vi "SudokuSolver.vi"() -> ()   [LabVIEW 2010]
uses:
  SudukuBoard/SudokuBoard.lvclass
  Graph/Graph.lvclass
panel:
  in  "Exit":bool
  in  "Solve":bool
  in  "Ultimate":bool
  in  "Hard":bool
  in  "Medium":bool
  in  "Easy":bool
  out "Board":T1(array[cluster])
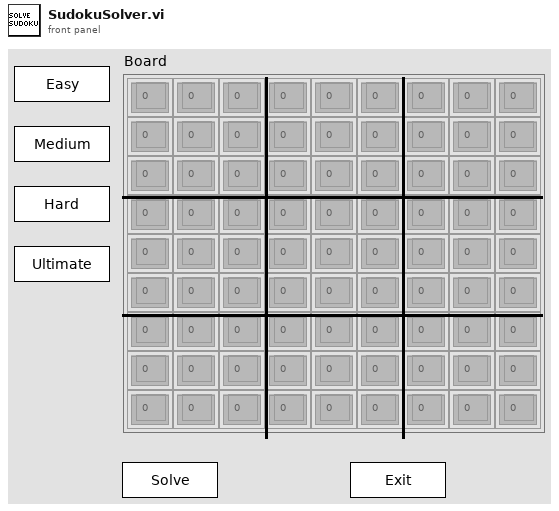
[diagram p1: front panel]
types:
  T1 = cluster{"dimension size":i32, "dimension size 2":bool}[][]
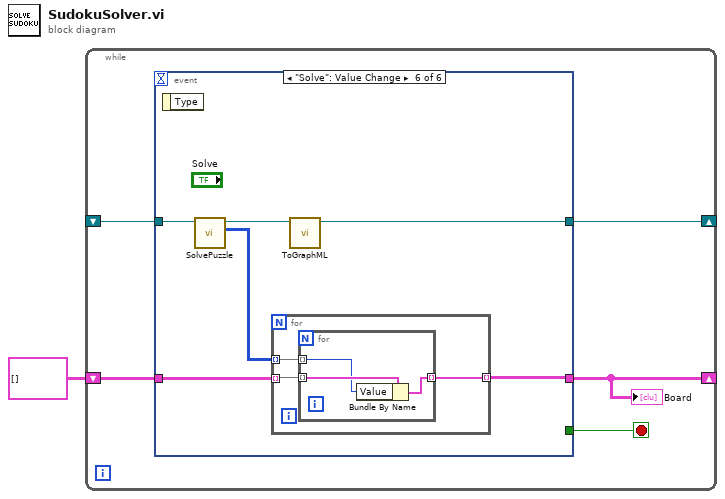
[diagram p0: block diagram]
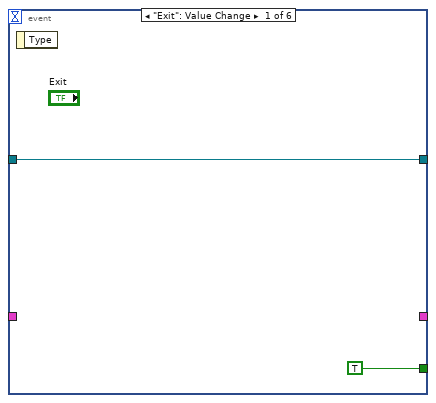
[diagram p2: hidden frame]
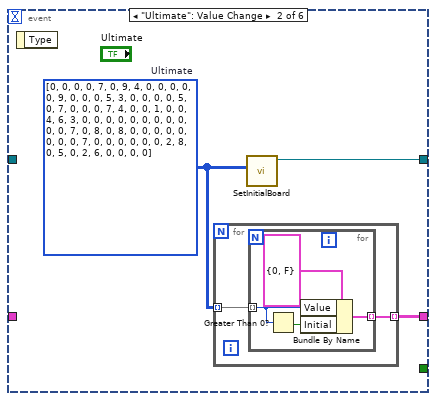
[diagram p3: hidden frame]
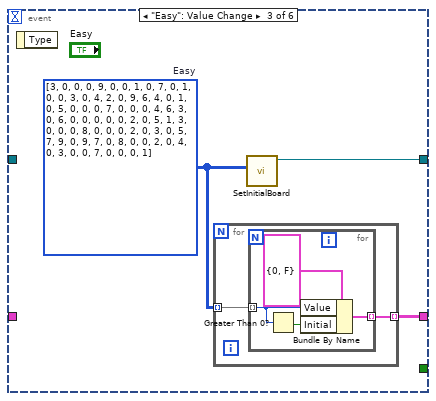
[diagram p4: hidden frame]
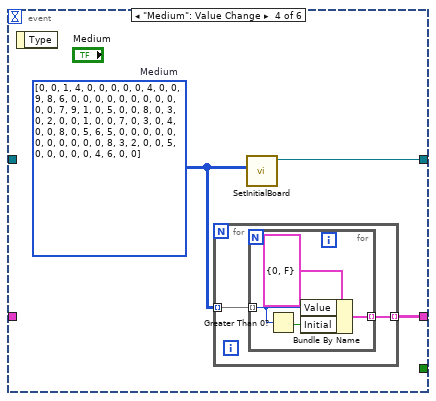
[diagram p5: hidden frame]
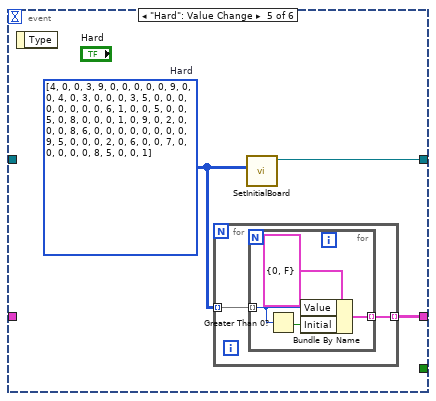
[diagram p6: hidden frame]
diagram:
  n1 = while {
    shift-right: [w5] -> _
    shift-left: _ -> [w4]
    shift-right: [w3] -> _
    shift-left: cluster{"Value":i32, "Initial":bool}[][] [] -> [w2]
    stop <- w6 stop-if-true
    n2 = event shown="[5] \"Solve\": Value Change" {
      selector: _ -> [_ _ _ _ _ _]
      dyn-events: _ -> [_ _ _ _ _ _]
      timeout: _ -> [_ _ _ _ _ _]
      tunnel: [TRUE _ _ _ _ _] -> w6
      tunnel: [w7 w11 w20 w29 w38 w45] -> w5
      tunnel: w4 -> [w7 _ _ _ _ w50]
      tunnel: [_ w9 w18 w28 w36 w47] -> w3
      tunnel: w2 -> [_ _ _ _ _ w49]
      event "Exit": Value Change {
        n3 = event-data() -> ()  [unwired: 1 in, 1 out]
      }
      event "Ultimate": Value Change {
        w10 = i32[][] [[0, 0, 0, 0, 7, 0, 9, 4, 0], [0, 0, 0, 0, 9, 0, 0, 0, 5], [3, 0, 0, 0, 0, 5, 0, 7, 0], [0, 0, 7, 4, 0, 0, 1, 0, 0], [4, 6, 3, 0, 0, 0, 0, 0, 0], [0, 0, 0, 0, 0, 7, 0, 8, 0], [8, 0, 0, 0, 0, 0, 0, 0, 0], [7, 0, 0, 0, 0, 0, 0, 2, 8], [0, 5, 0, 2, 6, 0, 0, 0, 0]]  # Ultimate
        n4 = event-data() -> ()  [unwired: 1 in, 1 out]
        n5 = for {
          tunnel: w10 -> [w13] mode=indexing
          tunnel: [w12] -> w9 mode=indexing
          n6 = for {
            tunnel: w13 -> [w16] mode=indexing
            tunnel: [w17] -> w12 mode=indexing
            n7 = Greater Than 0?(x=w16) -> (x > 0?=w14:bool)
            n8 = Bundle By Name(cluster=cluster{"Value":i32, "Initial":bool} {"Value"=0, "Initial"=FALSE} ("Cell"), "Value"=w16, "Initial"=w14) -> (w17:cluster{"Value":i32, "Initial":bool})
          }
        }
        n9 = call "SetInitialBoard.vi"("InitialBoard"=w10) -> ("SudukuBoard out"=w11:refnum<class "SudokuBoard.lvclass">)  [unwired: 9 in, 1 out]
      }
      event "Easy": Value Change {
        w19 = i32[][] [[3, 0, 0, 0, 9, 0, 0, 1, 0], [7, 0, 1, 0, 0, 3, 0, 4, 2], [0, 9, 6, 4, 0, 1, 0, 5, 0], [0, 0, 7, 0, 0, 0, 4, 6, 3], [0, 6, 0, 0, 0, 0, 0, 2, 0], [5, 1, 3, 0, 0, 0, 8, 0, 0], [0, 2, 0, 3, 0, 5, 7, 9, 0], [9, 7, 0, 8, 0, 0, 2, 0, 4], [0, 3, 0, 0, 7, 0, 0, 0, 1]]  # Easy
        n10 = event-data() -> ()  [unwired: 1 in, 1 out]
        n11 = for {
          tunnel: w19 -> [w22] mode=indexing
          tunnel: [w21] -> w18 mode=indexing
          n12 = for {
            tunnel: w22 -> [w25] mode=indexing
            tunnel: [w26] -> w21 mode=indexing
            n13 = Greater Than 0?(x=w25) -> (x > 0?=w23:bool)
            n14 = Bundle By Name(cluster=cluster{"Value":i32, "Initial":bool} {"Value"=0, "Initial"=FALSE} ("Cell"), "Value"=w25, "Initial"=w23) -> (w26:cluster{"Value":i32, "Initial":bool})
          }
        }
        n15 = call "SetInitialBoard.vi"("InitialBoard"=w19) -> ("SudukuBoard out"=w20:refnum<class "SudokuBoard.lvclass">)  [unwired: 9 in, 1 out]
      }
      event "Medium": Value Change {
        w27 = i32[][] [[0, 0, 1, 4, 0, 0, 0, 0, 0], [4, 0, 0, 9, 8, 6, 0, 0, 0], [0, 0, 0, 0, 0, 0, 0, 0, 7], [9, 1, 0, 5, 0, 0, 8, 0, 3], [0, 2, 0, 0, 1, 0, 0, 7, 0], [3, 0, 4, 0, 0, 8, 0, 5, 6], [5, 0, 0, 0, 0, 0, 0, 0, 0], [0, 0, 0, 8, 3, 2, 0, 0, 5], [0, 0, 0, 0, 0, 4, 6, 0, 0]]  # Medium
        n16 = event-data() -> ()  [unwired: 1 in, 1 out]
        n17 = for {
          tunnel: w27 -> [w31] mode=indexing
          tunnel: [w30] -> w28 mode=indexing
          n18 = for {
            tunnel: w31 -> [w34] mode=indexing
            tunnel: [w35] -> w30 mode=indexing
            n19 = Greater Than 0?(x=w34) -> (x > 0?=w32:bool)
            n20 = Bundle By Name(cluster=cluster{"Value":i32, "Initial":bool} {"Value"=0, "Initial"=FALSE} ("Cell"), "Value"=w34, "Initial"=w32) -> (w35:cluster{"Value":i32, "Initial":bool})
          }
        }
        n21 = call "SetInitialBoard.vi"("InitialBoard"=w27) -> ("SudukuBoard out"=w29:refnum<class "SudokuBoard.lvclass">)  [unwired: 9 in, 1 out]
      }
      event "Hard": Value Change {
        w37 = i32[][] [[4, 0, 0, 3, 9, 0, 0, 0, 0], [0, 9, 0, 0, 4, 0, 3, 0, 0], [0, 3, 5, 0, 0, 0, 0, 0, 0], [0, 0, 6, 1, 0, 0, 5, 0, 0], [5, 0, 8, 0, 0, 0, 1, 0, 9], [0, 2, 0, 0, 0, 8, 6, 0, 0], [0, 0, 0, 0, 0, 0, 9, 5, 0], [0, 0, 2, 0, 6, 0, 0, 7, 0], [0, 0, 0, 0, 8, 5, 0, 0, 1]]  # Hard
        n22 = event-data() -> ()  [unwired: 1 in, 1 out]
        n23 = for {
          tunnel: w37 -> [w40] mode=indexing
          tunnel: [w39] -> w36 mode=indexing
          n24 = for {
            tunnel: w40 -> [w43] mode=indexing
            tunnel: [w44] -> w39 mode=indexing
            n25 = Greater Than 0?(x=w43) -> (x > 0?=w41:bool)
            n26 = Bundle By Name(cluster=cluster{"Value":i32, "Initial":bool} {"Value"=0, "Initial"=FALSE} ("Cell"), "Value"=w43, "Initial"=w41) -> (w44:cluster{"Value":i32, "Initial":bool})
          }
        }
        n27 = call "SetInitialBoard.vi"("InitialBoard"=w37) -> ("SudukuBoard out"=w38:refnum<class "SudokuBoard.lvclass">)  [unwired: 9 in, 1 out]
      }
      event "Solve": Value Change {
        n28 = event-data() -> ()  [unwired: 1 in, 1 out]
        n29 = call "SolvePuzzle.vi"("Puzzle in"=w50) -> ("Solution"=w48:i32[][], "Puzzle out"=w46:refnum<class "SudokuBoard.lvclass">)  [unwired: 8 in, 1 out]
        n30 = for {
          tunnel: w48 -> [w53] mode=indexing
          tunnel: w49 -> [w52] mode=indexing
          tunnel: [w51] -> w47 mode=indexing
          n31 = for {
            tunnel: w53 -> [w55] mode=indexing
            tunnel: w52 -> [w56] mode=indexing
            tunnel: [w54] -> w51 mode=indexing
            n32 = Bundle By Name(cluster=w56, "Value"=w55) -> (w54:cluster{"Value":i32, "Initial":bool})
          }
        }
        n33 = call "ToGraphML.vi"("Graph in"=w46) -> ("Graph out"=w45:refnum<class "SudokuBoard.lvclass">)  [unwired: 9 in, 1 out]
      }
    }
    "Board" <- w3
  }
